vi "onMenuSelection.vi"(8 "error in (no error)":errorcluster, 10 "Item Tag":string, 11 "Filled Text Fields Actor in":refnum<class "Filled Text Fields Actor.lvclass">) -> (0 "error out":errorcluster, 3 "Filled Text Fields Actor out":refnum<class "Filled Text Fields Actor.lvclass">)   [LabVIEW 2017, in "Filled Text Fields.lvlib" / "Filled Text Fields Actor.lvclass"]
uses:
  Filled Text Fields Actor.lvclass
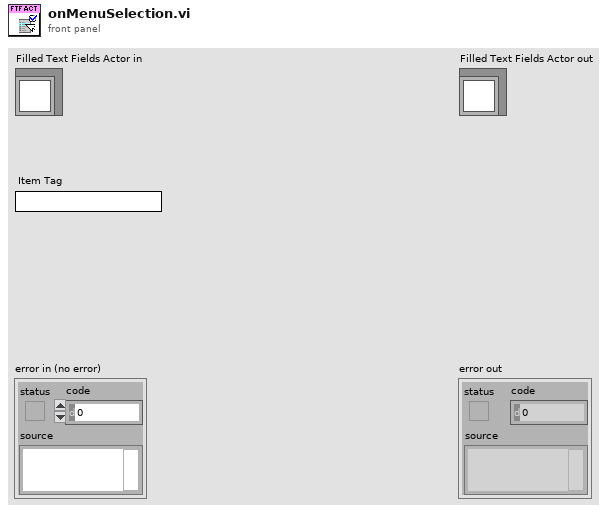
[diagram p1: front panel]
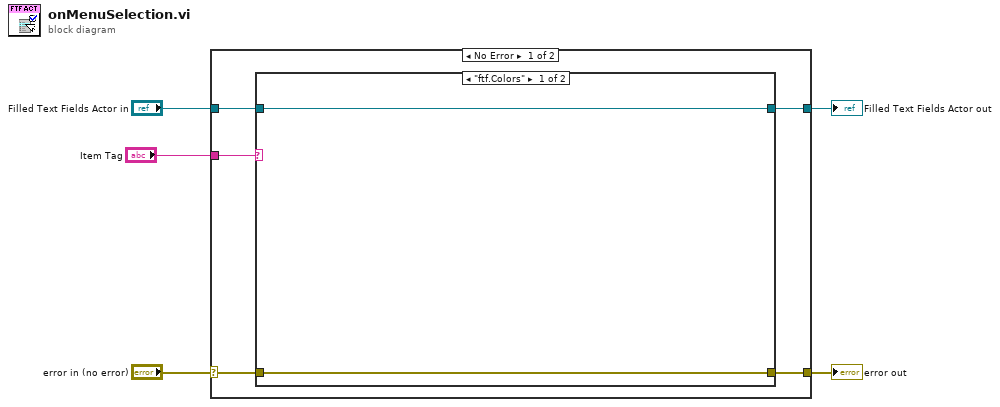
[diagram p0: block diagram]
diagram:
  n1 = case shown="No Error" "error in (no error)" {
    selector: "error in (no error)" -> [w8 w16]
    tunnel: [w7 w16] -> w4
    tunnel: [w6 w15] -> w2
    tunnel: "Filled Text Fields Actor in" -> [w9 w15]
    tunnel: "Item Tag" -> [w10 _]
    frame No Error {
      n2 = case shown="\"ftf.Colors\"" w10 {
        tunnel: w9 -> [w11 w13]
        tunnel: w8 -> [w12 w14]
        tunnel: [w12 w14] -> w7
        tunnel: [w11 w13] -> w6
        frame "ftf.Colors" {
        }
        frame Default {
        }
      }
    }
    frame Error {
    }
  }
  "error out" <- w4
  "Filled Text Fields Actor out" <- w2
